vi "Fetch (Measurements).vi"(0 "VISA resource name":refnum<visa-resource-name>, 5 "Timeout (10000 ms)":i32=10000 format="%#.6g", 11 "error in (no error)":errorcluster, 12 "ABORT?":bool) -> (3 "Voltage":sgl[](array[numeric]), 4 "VISA resource name out":refnum<visa-resource-name>, 6 "Current":sgl[](array[numeric]), 8 "Resistance":sgl[](array[numeric]), 10 "Timestamp":sgl[](array[numeric]), 14 "Status":sgl[](array[numeric]), 15 "error out":errorcluster)   [LabVIEW 2009, in "Keithley 24XX.lvlib"]
doc: "Fetches data for voltage, current, resistance, timestamp, and status. These readings are then provided in separate arrays for each type of reading.\n\n<B>Note</B> Use this VI only with other low-level VIs. The high-level VIs automatically incorporate this functionality. This VI does not check the instrument status. If you want to check the instrument status, call the Error Query VI at the conclusion of the sequence."
uses:
  Keithley 24XX.lvlib
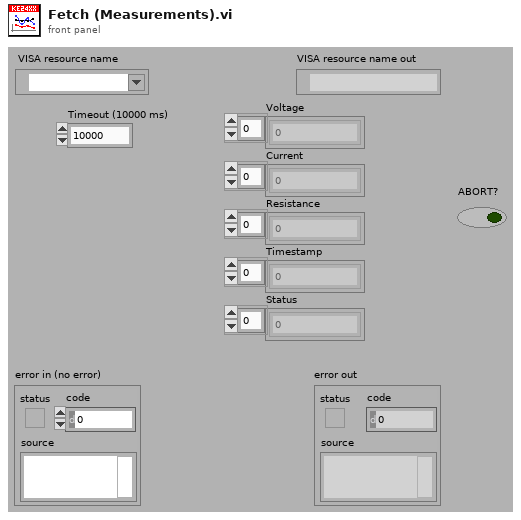
[diagram p1: front panel]
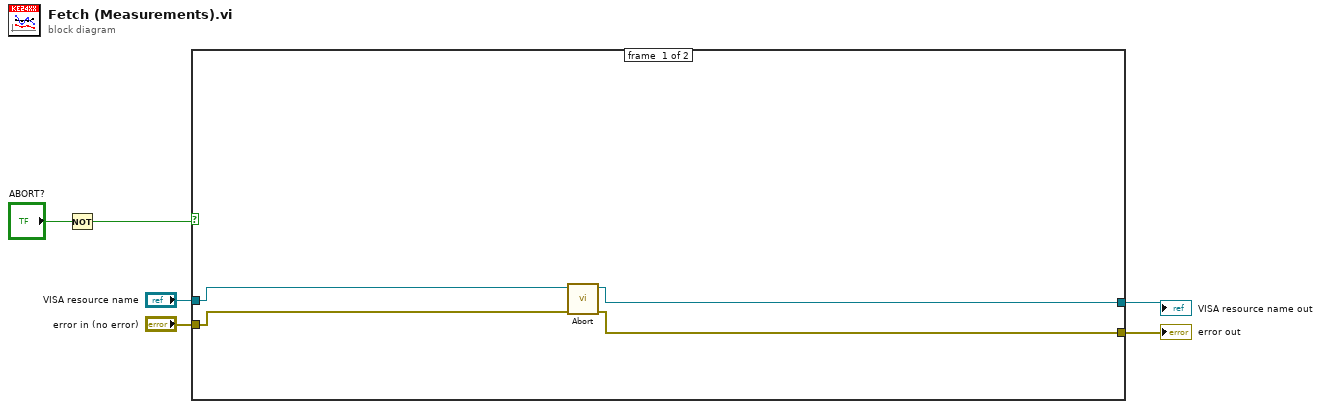
[diagram p0: block diagram]
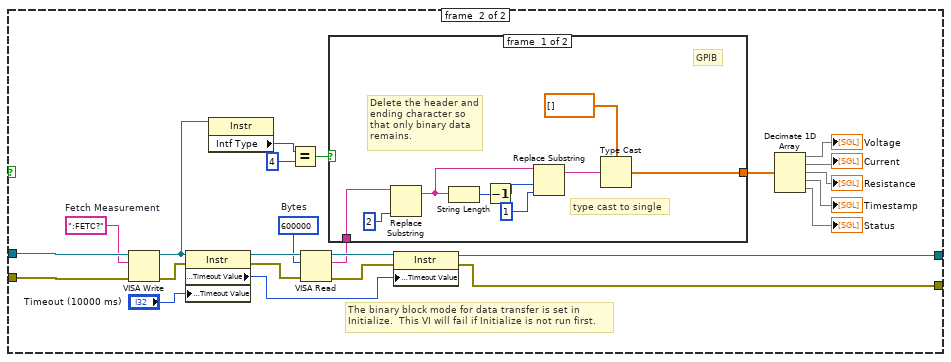
[diagram p2: hidden frame]
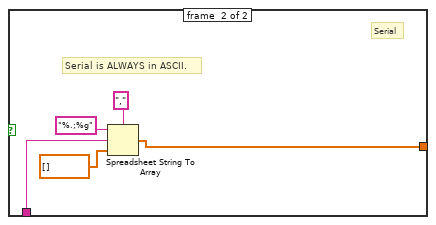
[diagram p3: hidden frame]
diagram:
  n1 = Not(x="ABORT?") -> (.not. x?=w1:bool)
  n2 = case shown="True" w1 {
    tunnel: "VISA resource name" -> [w10 w34]
    tunnel: "error in (no error)" -> [w9 w33]
    tunnel: [w8 w24] -> w4
    tunnel: [w7 w23] -> w3
    frame #0 {
      n3 = call "Abort.vi"("error in (no error)"=w9, "VISA resource name"=w10) -> ("error out"=w7:errorcluster, "VISA resource name out"=w8:refnum<visa-resource-name>)  [unwired: 8 out]
    }
    frame #1 {
      w32 = ":FETC?"  # Fetch Measurement
      w22 = u32 600000  # Bytes
      # "The binary block mode for data transfer is set in Initialize.  This VI will fail if Initialize is not run first."
      n4 = VISA Write(VISA resource name=w34, write buffer=w32, error in (no error)=w33) -> (VISA resource name out=w14:refnum<visa-resource-name>, error out=w31:errorcluster)  [unwired: 1 out]
      n5 = property class="Instr"(reference=w14, error in=w31, "General Settings:Timeout Value"="Timeout (10000 ms)") -> (reference out=w30:refnum<visa-resource-name>, error out=w29:errorcluster, "General Settings:Timeout Value"=w25:u32)
      n6 = property class="Instr"(reference=w14) -> ("Intf Type"=w13:u16)  [unwired: 1 in, 2 out]
      n7 = Equal?(x=w13, y=u16 4) -> (x = y?=w11:bool)
      n8 = VISA Read(VISA resource name=w30, byte count=w22, error in (no error)=w29) -> (VISA resource name out=w27:refnum<visa-resource-name>, read buffer=w21:string, error out=w26:errorcluster)  [unwired: 1 out]
      n9 = case shown="False" w11 {
        tunnel: w21 -> [w43 w44]
        tunnel: [w36 w45] -> w20
        frame #0 {
          # "Delete the header and ending character so that only binary data remains."
          # "GPIB"
          # "type cast to single"
          n10 = Replace Substring(2:2 ("length (len. of substring)"), 5:w43) -> (1:w41:string)  [unwired: 3 out]
          n11 = String Length(string=w41) -> (length=w40:i32)
          n12 = Decrement(x=w40) -> (x-1=w39:i32)
          n13 = Replace Substring(2:1 ("length (len. of substring)"), 3:w39, 5:w41) -> (1:w35:string)  [unwired: 2 out]
          n14 = Type Cast(type=sgl[] [], x=w35) -> (*(type *) &x=w36:sgl[])
        }
        frame #1 {
          # "Serial is ALWAYS in ASCII."
          # "Serial"
          n15 = Spreadsheet String To Array(delimiter (Tab)=",", format string="%.;%g", spreadsheet string=w44, array type (2D Dbl)=sgl[] []) -> (array=w45:sgl[])
        }
      }
      n16 = property class="Instr"(reference=w27, error in=w26, "General Settings:Timeout Value"=w25) -> (reference out=w24:refnum<visa-resource-name>, error out=w23:errorcluster)
      n17 = Decimate 1D Array(w20) -> (→"Voltage":sgl[], →"Current":sgl[], →"Resistance":sgl[], →"Timestamp":sgl[], →"Status":sgl[])
    }
  }
  "error out" <- w3
  "VISA resource name out" <- w4
